vi "App_Main Stop.vi"(8 "error in":errorcluster) -> (0 "error out":errorcluster)   [LabVIEW 2015, in "Application 2.lvlib"]
uses:
  Application 2.lvlib
  Data Def/App_Subpanel Name.ctl
  Data Def/App_User Event Data.ctl
  Data Def/App_Main Loop Queue Data.ctl
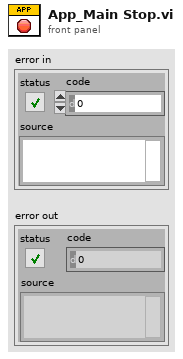
[diagram p1: front panel]
types:
  T1 = typedef "Application 2.lvlib/App_Main Loop Queue Data.ctl" = cluster{"Command":string, "Data":variant}
  T2 = typedef "Application 2.lvlib/App_User Event Data.ctl" = cluster{"Command":string, "Data":variant}
  T3 = typedef "Application 2.lvlib/App_Subpanel Name.ctl" = enum16{"Main", "Menu", "User Registering", "User Setting", "Monitor", "Traning Mode", "Query Data", "Connect Setting"}
  T4 = typedef "Application 2.lvlib/App_Main Data.ctl" = cluster{"VI Refnum":refnum<vi>, "Subpanel":refnum<vi>, "Connection ID":refnum<k5>, "Meta data":T5[], "Main Queue":T7, "User Data":T8}
  T5 = typedef "stm_MetaElement.ctl" = cluster{"Name":T6}
  T6 = typedef "stm_MetaDataElement.ctl" = string
  T7 = typedef "Application 2.lvlib/App_Main Queue.ctl" = cluster{"Main Loop Queue":refnum<queue>}
  T8 = typedef "User Data.ctl" = cluster{"Name":string, "Email":string, "Phone Number":string, "User Picture":u32[][], "Last Login Time":timestamp}
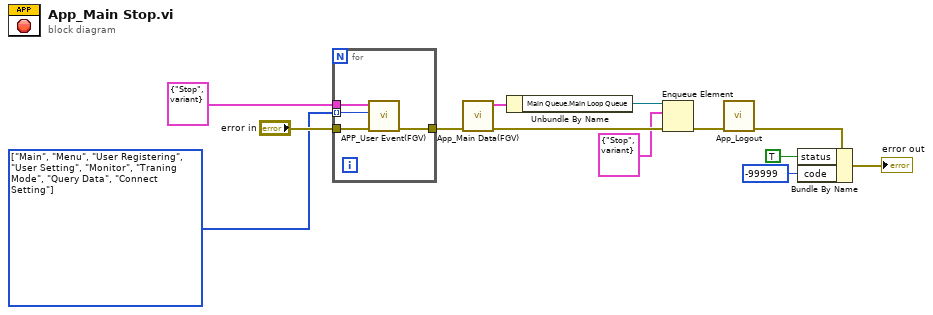
[diagram p0: block diagram]
diagram:
  w12 = T3[] [enum."Main", enum."Menu", enum."User Registering", enum."User Setting", enum."Monitor", enum."Traning Mode", enum."Query Data", enum."Connect Setting"] items=["Main", "Menu", "User Registering", "User Setting", "Monitor", "Traning Mode", "Query Data", "Connect Setting"] ("Array")
  n1 = for {
    tunnel: "error in" -> [w17]
    tunnel: w12 -> [w16] mode=indexing
    tunnel: [w15] -> w7
    tunnel: T2 {"Command"="Stop", "Data"=variant} ("User Event Data") -> [w14]
    n2 = call "APP_User Event(FGV).vi"("error in"=w17, "Subpanel Name"=w16, "User Event Data"=w14) -> ("error out"=w15:errorcluster)  [unwired: 7 in, 1 out]
  }
  n3 = call "App_Main Data(FGV).vi"("error in"=w7) -> ("error out"=w6:errorcluster, "Main Data Out"=w8:T4)  [unwired: 9 in]
  n4 = Unbundle By Name(w8) -> ("Main Queue.Main Loop Queue"=w5:refnum<queue>)
  n5 = Enqueue Element(queue=w5, element=T1 {"Command"="Stop", "Data"=variant}, error in (no error)=w6) -> (error out=w2:errorcluster)  [unwired: 1 in, 2 out]
  n6 = call "App_Logout.vi"("error in"=w2) -> ("error out"=w1:errorcluster)  [unwired: 10 in]
  n7 = Bundle By Name(cluster=w1, "status"=TRUE, "code"=-99999) -> (→"error out":errorcluster)
